vi "Write PV Data Queue.vi"(8 "error in (no error)":errorcluster, 10 "Data Queue":refnum<queue>, 11 "CS++DIMMonitor in":refnum<class "CS++DIMMonitor.lvclass">) -> (0 "error out":errorcluster, 3 "CS++DIMMonitor out":refnum<class "CS++DIMMonitor.lvclass">)   [LabVIEW 2016, in "CS++DIMMonitor.lvlib" / "CS++DIMMonitor.lvclass"]
doc: "Set PV command/service data queue.\n\nThis VI was introduced because of DIM."
uses:
  CS++DIMMonitor.lvclass
  CS++DIMMonitor.lvclass/CS++DIMMonitor.ctl
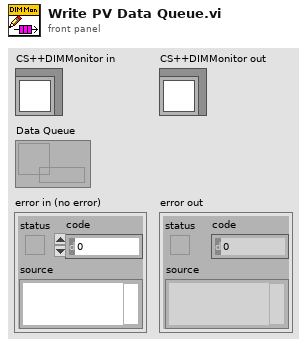
[diagram p1: front panel]
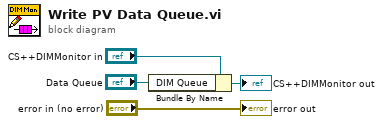
[diagram p0: block diagram]
diagram:
  n1 = Bundle By Name(cluster="CS++DIMMonitor in", "DIM Queue"="Data Queue") -> (→"CS++DIMMonitor out":refnum<class "CS++DIMMonitor.lvclass">)
  "error out" <- "error in (no error)"
